vi "TDMSAddBlankElem2d.vi"(1 "input 2d string array":string[][](array[string])) -> (0 "output 2d string array with the first column blank":string[][](array[string]))   [LabVIEW 2017]
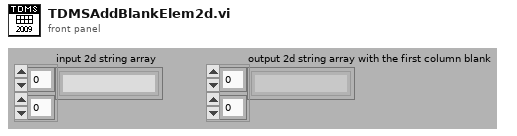
[diagram p1: front panel]
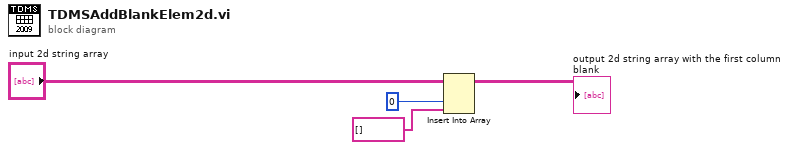
[diagram p0: block diagram]
diagram:
  n1 = Insert Into Array(array="input 2d string array", index (col)=0 ("disabled index (col)"), new element=string[] [] ("new element/subarray")) -> (→"output 2d string array with the first column blank":string[][])  [unwired: 1 in]
